vi "4Pi Obj Lock - Setup Camera.vi"(0 "Camera Notifier Name":string) -> (8 "Canceled?":bool)   [LabVIEW 2016]
uses:
  <vilib>/Utility/miscctls.llb/LVPointTypeDef.ctl
  Device Library/Cameras/Camera Controls/Generic Camera ROI.ctl
  Device Library/Cameras/Camera Controls/Generic Camera Actions.ctl
  4Pi Objective Lock Type Defs/4Pi Obj Lock - Camera Settings.ctl
panel:
  out "ROI Size":string
  in  "Exposure Time (ms)":dbl
  in  "Tool Selection":enum32{"Zoom Tool", "ROI Tool", "Pan Tool"}(radio)
  in  "Cancel":bool
  in  "Done":bool
  out "Camera Display":T1(plugin-control)
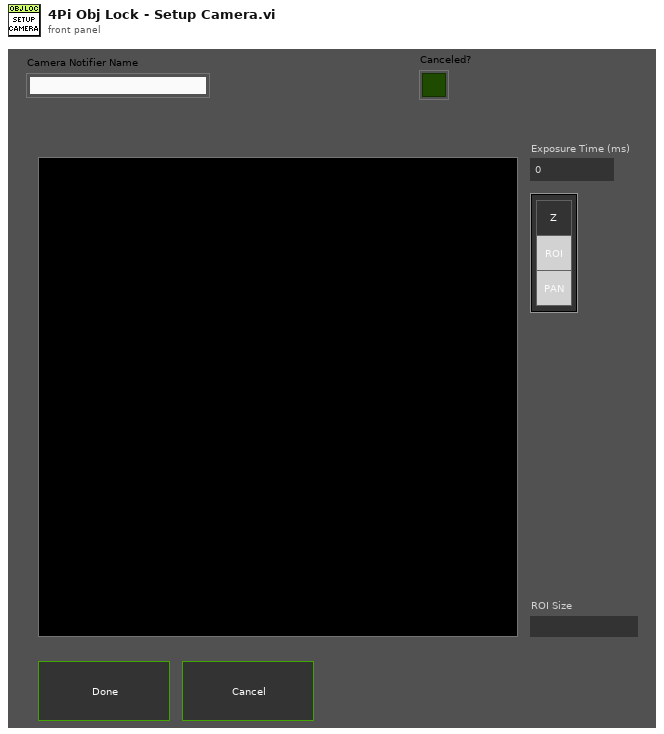
[diagram p1: front panel]
types:
  T1 = typedef "IMAQ Image.ctl" = refnum<image>
  T2 = typedef "Generic Camera Actions.ctl" = enum16{"Status", "Live Preview", "Capture", "Abort", "Set Exposure Time (s)", "Get Exposure Time (s)", "Record Settings", "Set ROI", "Get ROI", "Defect Correction On/Off", "Cooler On/Off", "Fan On/Off", "Quit"}
  T3 = typedef "Generic Camera ROI.ctl" = cluster{"H_Offset":u16, "V_Offset":u16, "H_Width":u16, "V_Width":u16}
  T4 = enum16{"Always On", "Always Off", "Off While Running"}
  T5 = typedef "LVPointTypeDef.ctl" = cluster{"Horizontal":i16, "Vertical":i16}
  T6 = typedef "LVRectTypeDef.ctl" = cluster{"Left":i16, "Top":i16, "Right":i16, "Bottom":i16}
  T7 = typedef "LVBoundsTypeDef.ctl" = cluster{"Width":u32, "Height":u32}
  T8 = typedef "4Pi Obj Lock - Camera Settings.ctl" = cluster{"Exposure Time (s)":dbl, "H Offset":u16, "V Offset":u16, "H Width":u16, "V Width":u16}
  T9 = cluster{"Global Rectangle":i32[], "Contours":cluster{"Contour Type":u32, "ROI Type":u32, "Points":i32[]}[]}
  T10 = cluster{"Contour Type":u32, "ROI Type":u32, "Points":i32[]}[]
  T11 = cluster{"Contour Type":u32, "ROI Type":u32, "Points":i32[]}
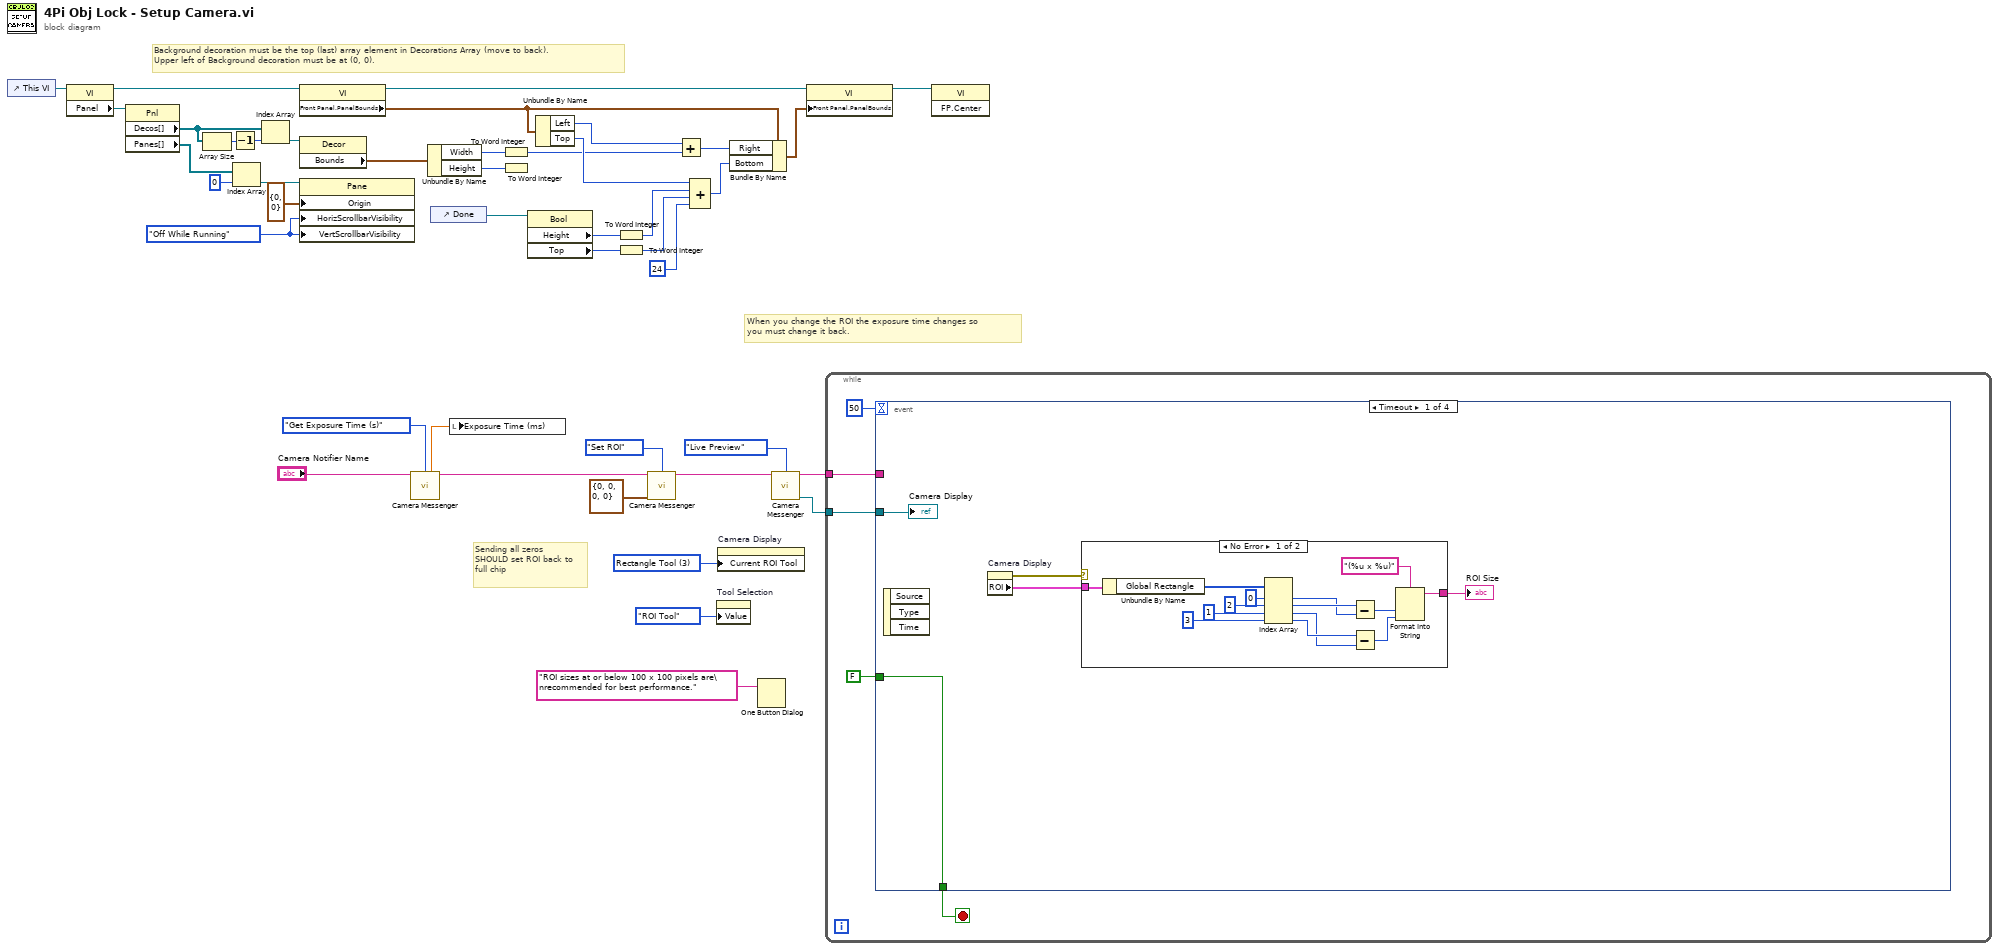
[diagram p0: block diagram]
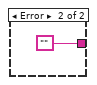
[diagram p2: hidden frame]
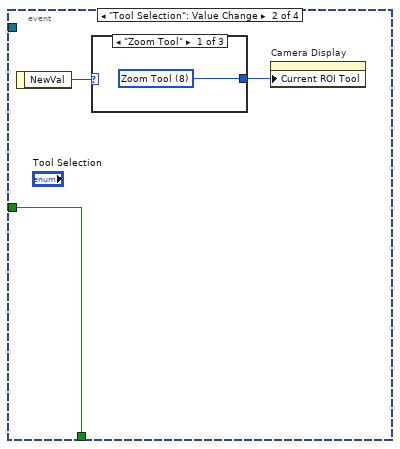
[diagram p3: hidden frame]
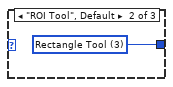
[diagram p4: hidden frame]
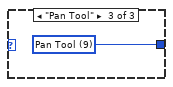
[diagram p5: hidden frame]
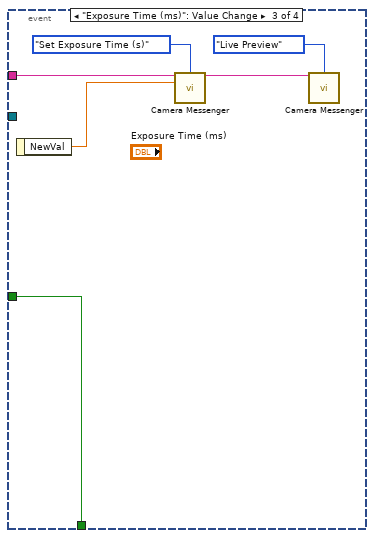
[diagram p6: hidden frame]
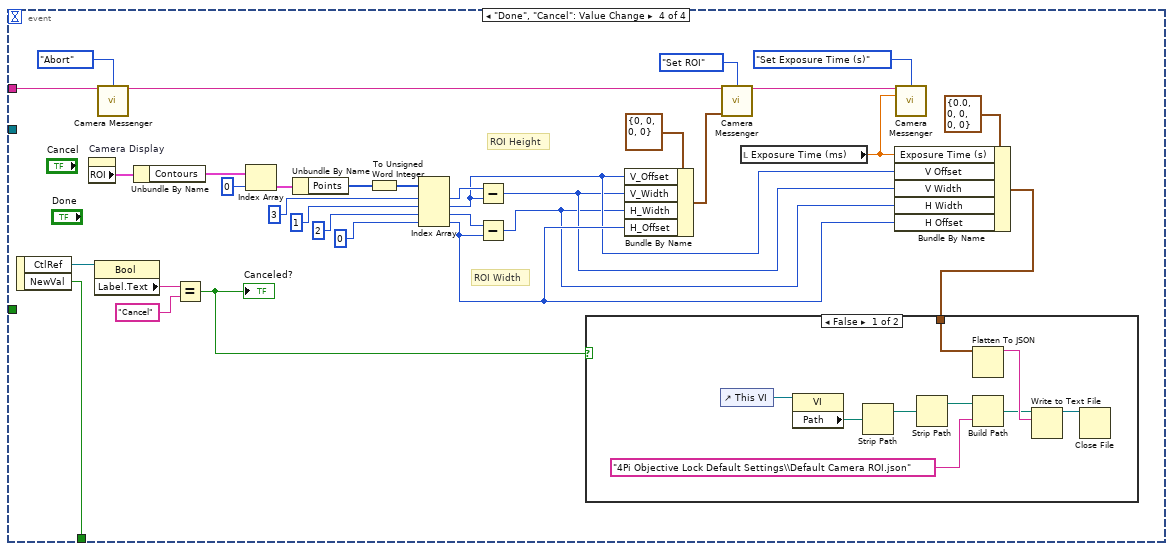
[diagram p7: hidden frame]
diagram:
  w24 = T4."Off While Running" ("Vertical Scrollbar Visibility")
  w43 = u32 3 items=["Zoom Tool"=8, "Selection Tool"=0, "Pan Tool"=9, "Point Tool"=1, "Line Tool"=2, "Rectangle Tool"=3, "Rotated Rectangle Tool"=12, "Polyline Tool"=10, "Polygon Tool"=5, "Freehand Tool"=11, "Closed Freehand Tool"=6, "Ellipse Tool"=4, "Annulus Tool"=7] ("Current ROI Tool")
  # "Background decoration must be the top (last) array element in Decorations Array (move to back).\nUpper left of Background decoration must be at (0, 0)."
  # "When you change the ROI the exposure time changes so\nyou must change it back."
  # "Sending all zeros SHOULD set ROI back to full chip"
  n1 = control-ref of="This VI"() -> (w16:refnum<vi>)
  n2 = property class="VI"(reference=w16) -> (reference out=w25:refnum<vi>, "Panel"=w17:refnum<vi>)  [unwired: 1 in, 1 out]
  n3 = property class="Pnl"(reference=w17) -> ("Decos[]"=w15:refnum<vi>[], "Panes[]"=w21:refnum<vi>[])  [unwired: 1 in, 2 out]
  n4 = Array Size(array=w15) -> (size(s)=w13:i32)
  n5 = Decrement(x=w13) -> (x-1=w14:i32)
  n6 = Index Array(array=w21, index=0) -> (element=w20:refnum<vi>)
  n7 = Index Array(array=w15, index=w14) -> (element=w23:refnum<vi>)
  n8 = property class="VI"(reference=w25) -> (reference out=w27:refnum<vi>, "Front Panel.PanelBounds"=w28:T6)  [unwired: 1 in, 1 out]
  n9 = property class="Decor"(reference=w23) -> ("Bounds"=w26:T7)  [unwired: 1 in, 2 out]
  n10 = property class="Pane"(reference=w20, "Origin"=T5 {"Horizontal"=0, "Vertical"=0}, "HorizScrollbarVisibility"=w24, "VertScrollbarVisibility"=w24) -> ()  [unwired: 1 in, 2 out]
  n11 = call "Camera Messenger.vi"("Notifier Name"="Camera Notifier Name", "General Camera Actions"=Generic_Camera_Actions."Get Exposure Time (s)") -> ("Current Exposure Time (s)"=w9:dbl, "Notifier Name Dup"=w8:string)  [unwired: 8 in, 4 out]
  n12 = Unbundle By Name(w26) -> ("Width"=w31:u32, "Height"=w34:u32)
  n13 = control-ref of="Done"() -> (w18:refnum<vi>)
  n14 = local write "Exposure Time (ms)"(w9) -> ()
  n15 = To Word Integer(number=w31) -> (16bit integer=w33:i16)
  n16 = To Word Integer(number=w34) -> ()  [unwired: 1 out]
  n17 = property class="Bool"(reference=w18) -> ("Height"=w36:u32, "Top"=w37:i32)  [unwired: 1 in, 2 out]
  n18 = Unbundle By Name(w28) -> ("Left"=w30:i16, "Top"=w41:i16)
  n19 = To Word Integer(number=w36) -> (16bit integer=w39:i16)
  n20 = To Word Integer(number=w37) -> (16bit integer=w40:i16)
  n21 = call "Camera Messenger.vi"("Notifier Name"=w8, "General Camera Actions"=Generic_Camera_Actions."Set ROI", "Camera ROI"=T3 {"H_Offset"=0, "V_Offset"=0, "H_Width"=0, "V_Width"=0} ("General Camera ROI")) -> ("Notifier Name Dup"=w5:string)  [unwired: 7 in, 5 out]
  n22 = Add(x=w30, y=w33) -> (x+y=w32:i16)
  n23 = Compound Arithmetic op=ADD(w41, w39, w40, i16 24 ("y")) -> (w35:i16)
  n24 = property on="Tool Selection" class="RadioBtnsControl (strict)"("Value"=enum32{"Zoom Tool", "ROI Tool", "Pan Tool"}."ROI Tool" ("Tool Selection")) -> ()  [unwired: 2 in, 2 out]
  n25 = property on="Camera Display" class="ImageControl"("Current ROI Tool"=w43) -> ()  [unwired: 2 in, 2 out]
  n26 = Bundle By Name(cluster=w28, "Right"=w32, "Bottom"=w35) -> (w29:T6)
  n27 = One Button Dialog(message="ROI sizes at or below 100 x 100 pixels are\nrecommended for best performance.") -> ()  [unwired: 1 in, 1 out]
  n28 = call "Camera Messenger.vi"("Notifier Name"=w5, "General Camera Actions"=Generic_Camera_Actions."Live Preview") -> ("Notifier Name Dup"=w4:string, "Image Ref"=w2:T1)  [unwired: 8 in, 4 out]
  n29 = property class="VI"(reference=w27, "Front Panel.PanelBounds"=w29) -> (reference out=w12:refnum<vi>)  [unwired: 1 in, 1 out]
  n30 = while {
    tunnel: w2 -> [w46]
    tunnel: w4 -> [w44]
    stop <- w48 stop-if-true
    n31 = event shown="[0] Timeout" {
      selector: _ -> [_ _ _ _]
      dyn-events: _ -> [_ _ _ _]
      timeout: 50 -> [_ _ _ _]
      tunnel: [w53 w71 w80 w109] -> w48
      tunnel: FALSE -> [w53 w71 w80 _]
      tunnel: w46 -> [w52 _ _ _]
      tunnel: w44 -> [_ _ w79 w97]
      event Timeout {
        n32 = event-data() -> ()  [unwired: 1 in, 3 out]
        n33 = property on="Camera Display" class="ImageControl"() -> (error out=w50:errorcluster, "ROI"=w51:T9)  [unwired: 2 in, 1 out]
        n34 = case shown="No Error" w50 {
          tunnel: w51 -> [w58 _]
          tunnel: [w54 ""] -> w49
          frame No Error {
            n35 = Unbundle By Name(w58) -> ("Global Rectangle"=w67:i32[])
            n36 = Index Array(array=w67, index #1=0 ("index"), index #2=2 ("index"), index #3=1 ("index"), index #4=3 ("index")) -> (element #1=w61:i32, element #2=w62:i32, element #3=w59:i32, element #4=w60:i32)
            n37 = Subtract(x=w62, y=w61) -> (x-y=w56:i32)
            n38 = Subtract(x=w60, y=w59) -> (x-y=w55:i32)
            n39 = Format Into String(format string="(%u x %u)", w56, w55) -> (resulting string=w54:string)  [unwired: 2 in, 1 out]
          }
          frame Error {
          }
        }
        "ROI Size" <- w49
        "Camera Display" <- w52
      }
      event "Tool Selection": Value Change {
        n40 = event-data() -> ("NewVal"=w70:enum32{"Zoom Tool", "ROI Tool", "Pan Tool"})  [unwired: 1 in]
        n41 = case shown="\"Zoom Tool\"" w70 {
          tunnel: [w72 w73 w74] -> w69
          frame "Zoom Tool" {
            w72 = u32 8 items=["Zoom Tool"=8, "Selection Tool"=0, "Pan Tool"=9, "Point Tool"=1, "Line Tool"=2, "Rectangle Tool"=3, "Rotated Rectangle Tool"=12, "Polyline Tool"=10, "Polygon Tool"=5, "Freehand Tool"=11, "Closed Freehand Tool"=6, "Ellipse Tool"=4, "Annulus Tool"=7] ("Current ROI Tool")
          }
          frame "ROI Tool", Default {
            w73 = u32 3 items=["Zoom Tool"=8, "Selection Tool"=0, "Pan Tool"=9, "Point Tool"=1, "Line Tool"=2, "Rectangle Tool"=3, "Rotated Rectangle Tool"=12, "Polyline Tool"=10, "Polygon Tool"=5, "Freehand Tool"=11, "Closed Freehand Tool"=6, "Ellipse Tool"=4, "Annulus Tool"=7] ("Current ROI Tool")
          }
          frame "Pan Tool" {
            w74 = u32 9 items=["Zoom Tool"=8, "Selection Tool"=0, "Pan Tool"=9, "Point Tool"=1, "Line Tool"=2, "Rectangle Tool"=3, "Rotated Rectangle Tool"=12, "Polyline Tool"=10, "Polygon Tool"=5, "Freehand Tool"=11, "Closed Freehand Tool"=6, "Ellipse Tool"=4, "Annulus Tool"=7] ("Current ROI Tool")
          }
        }
        n42 = property on="Camera Display" class="ImageControl"("Current ROI Tool"=w69) -> ()  [unwired: 2 in, 2 out]
      }
      event "Exposure Time (ms)": Value Change {
        n43 = event-data() -> ("NewVal"=w77:dbl)  [unwired: 1 in]
        n44 = call "Camera Messenger.vi"("Notifier Name"=w79, "General Camera Actions"=Generic_Camera_Actions."Set Exposure Time (s)", "Exposure Time (s)"=w77) -> ("Notifier Name Dup"=w76:string)  [unwired: 7 in, 5 out]
        n45 = call "Camera Messenger.vi"("Notifier Name"=w76, "General Camera Actions"=Generic_Camera_Actions."Live Preview") -> ()  [unwired: 8 in, 6 out]
      }
      event "Done", "Cancel": Value Change {
        # "ROI Width"
        # "ROI Height"
        n46 = event-data() -> ("CtlRef"=w112:refnum<vi>, "NewVal"=w109:bool)  [unwired: 1 in]
        n47 = property on="Camera Display" class="ImageControl"() -> ("ROI"=w105:T9)  [unwired: 2 in, 2 out]
        n48 = property class="Bool"(reference=w112) -> ("Label.Text"=w111:string)  [unwired: 1 in, 2 out]
        n49 = call "Camera Messenger.vi"("Notifier Name"=w97, "General Camera Actions"=Generic_Camera_Actions."Abort") -> ("Notifier Name Dup"=w94:string)  [unwired: 8 in, 5 out]
        n50 = Unbundle By Name(w105) -> ("Contours"=w104:T10)
        n51 = Equal?(x=w111, y="Cancel") -> (x = y?=w81:bool)
        "Canceled?" <- w81
        n52 = Index Array(array=w104, index=0) -> (element=w103:T11)
        n53 = Unbundle By Name(w103) -> ("Points"=w106:i32[])
        n54 = To Unsigned Word Integer(number=w106) -> (unsigned 16bit integer=w87:u16[])
        n55 = Index Array(array=w87, index #1=3 ("index"), index #2=1 ("index"), index #3=2 ("index"), index #4=0 ("index")) -> (element #1=w108:u16, element #2=w85:u16, element #3=w107:u16, element #4=w86:u16)
        n56 = Subtract(x=w108, y=w85) -> (x-y=w84:u16)
        n57 = Subtract(x=w107, y=w86) -> (x-y=w83:u16)
        n58 = Bundle By Name(cluster=T3 {"H_Offset"=0, "V_Offset"=0, "H_Width"=0, "V_Width"=0} ("General Camera ROI"), "V_Offset"=w85, "V_Width"=w84, "H_Width"=w83, "H_Offset"=w86) -> (w93:T3)
        n59 = call "Camera Messenger.vi"("Notifier Name"=w94, "General Camera Actions"=Generic_Camera_Actions."Set ROI", "Camera ROI"=w93) -> ("Notifier Name Dup"=w91:string)  [unwired: 7 in, 5 out]
        n60 = local read "Exposure Time (ms)"() -> (w88:dbl)
        n61 = Bundle By Name(cluster=T8 {"Exposure Time (s)"=0.0, "H Offset"=0, "V Offset"=0, "H Width"=0, "V Width"=0} ("Camera Settings"), "Exposure Time (s)"=w88, "V Offset"=w85, "V Width"=w84, "H Width"=w83, "H Offset"=w86) -> (w82:T8)
        n62 = case shown="False" w81 {
          tunnel: w82 -> [w113 _]
          frame False {
            n63 = control-ref of="This VI"() -> (w116:refnum<vi>)
            n64 = property class="VI"(reference=w116) -> ("Path"=w115:path)  [unwired: 1 in, 2 out]
            n65 = Strip Path(path=w115) -> (stripped path=w117:path)  [unwired: 1 out]
            n66 = Strip Path(path=w117) -> (stripped path=w118:path)  [unwired: 1 out]
            n67 = Flatten To JSON(anything=w113) -> (JSON string=w120:string)  [unwired: 2 in, 1 out]
            n68 = Build Path(base path=w118, name or relative path="4Pi Objective Lock Default Settings\\Default Camera ROI.json") -> (appended path=w114:path)
            n69 = Write to Text File(file (use dialog)=w114, text=w120) -> (refnum out=w121:refnum<file>)  [unwired: 2 in, 2 out]
            n70 = Close File(refnum=w121) -> ()  [unwired: 1 in, 2 out]
          }
          frame True {
          }
        }
        n71 = call "Camera Messenger.vi"("Notifier Name"=w91, "General Camera Actions"=Generic_Camera_Actions."Set Exposure Time (s)", "Exposure Time (s)"=w88) -> ()  [unwired: 7 in, 6 out]
      }
    }
  }
  n72 = invoke class="VI" method="FP.Center"(reference=w12) -> ()  [unwired: 2 in, 3 out]
